vi "Update Tree Height.vi"(11 "Settings UI in":refnum<class "Settings UI.lvclass">) -> (3 "Settings UI out":refnum<class "Settings UI.lvclass">)   [LabVIEW 2020, in "Output Sequencer.lvlib" / "Settings UI.lvclass"]
uses:
  Settings UI.lvclass
  Settings UI.lvclass/Settings UI.ctl
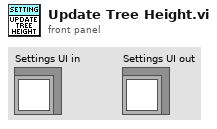
[diagram p1: front panel]
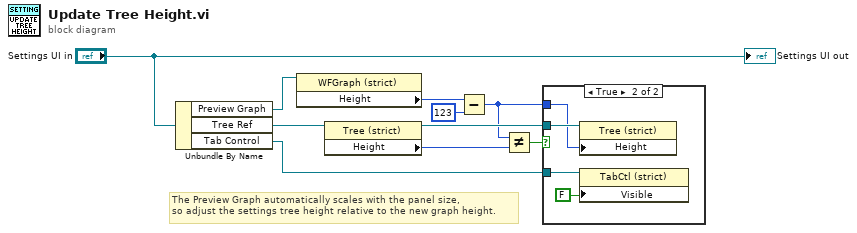
[diagram p0: block diagram]
diagram:
  # "The Preview Graph automatically scales with the panel size,\nso adjust the settings tree height relative to the new graph height."
  n1 = Unbundle By Name("Settings UI in") -> ("Preview Graph"=w5:refnum<vi>, "Tree Ref"=w4:refnum<vi>, "Tab Control"=w2:refnum<vi>)
  n2 = property on="Property Node" class="WFGraph (strict)"(reference=w5) -> ("Height"=w9:u32)  [unwired: 1 in, 2 out]
  n3 = property on="Property Node" class="Tree (strict)"(reference=w4) -> (reference out=w3:refnum<vi>, "Height"=w7:u32)  [unwired: 1 in, 1 out]
  n4 = Subtract(x=w9, y=u32 123) -> (x-y=w1:u32)
  n5 = Not Equal?(x=w1, y=w7) -> (x != y?=w6:bool)
  n6 = case shown="True" w6 {
    tunnel: w3 -> [_ w13]
    tunnel: w2 -> [_ w12]
    tunnel: w1 -> [_ w11]
    frame False {
    }
    frame True {
      n7 = property on="Property Node" class="Tree (strict)"(reference=w13, "Height"=w11) -> ()  [unwired: 1 in, 2 out]
      n8 = property on="Property Node" class="TabCtl (strict)"(reference=w12, "Visible"=FALSE) -> ()  [unwired: 1 in, 2 out]
    }
  }
  "Settings UI out" <- "Settings UI in"
